vi "Construct Message Counts Executions.vi"(8 "error in (no error)":errorcluster) -> (0 "error out":errorcluster, 2 "Message Executions":refnum<notifier>, 3 "CyclicMessageCountsCycles out":refnum<class "MessageCountsExecutions.lvclass">)   [LabVIEW 2017, in "MessageCountsExecutions.lvclass"]
uses:
  MessageCountsExecutions.lvclass
  MessageCountsExecutions.lvclass/MessageCountsExecutions.ctl
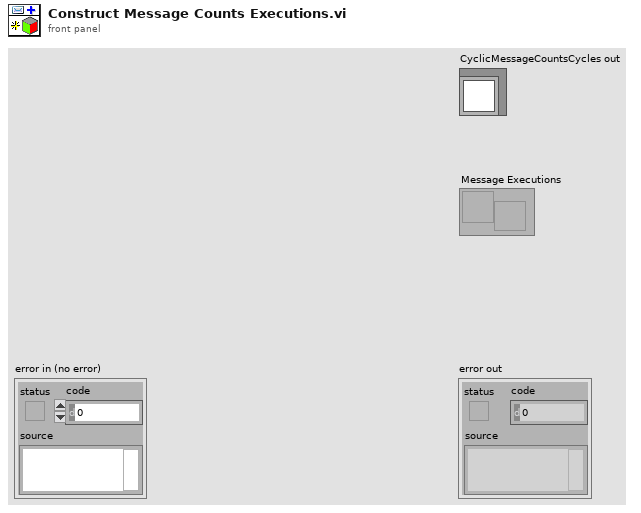
[diagram p1: front panel]
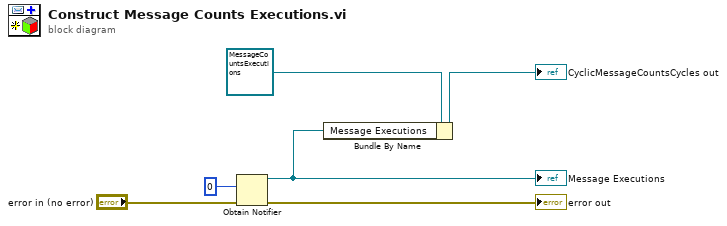
[diagram p0: block diagram]
diagram:
  n1 = Obtain Notifier(notification data type=u32 0, error in (no error)="error in (no error)") -> (notifier out=w1:refnum<notifier>, error out=→"error out":errorcluster)  [unwired: 2 in, 1 out]
  "Message Executions" <- w1
  n2 = Bundle By Name(cluster=refnum<class "MessageCountsExecutions.lvclass"> refnum ("CyclicMessageCountsCycles in"), "Message Executions"=w1) -> (→"CyclicMessageCountsCycles out":refnum<class "MessageCountsExecutions.lvclass">)
